vi "Enter_temp_sub_panel.vi"() -> ()   [LabVIEW 2011]
panel:
  in  "Stop":bool
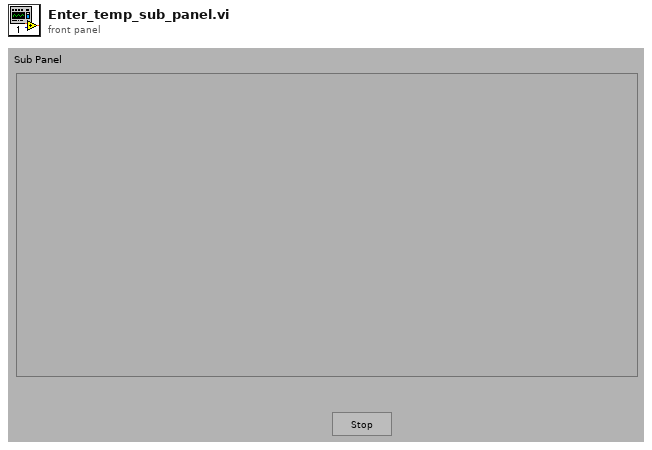
[diagram p1: front panel]
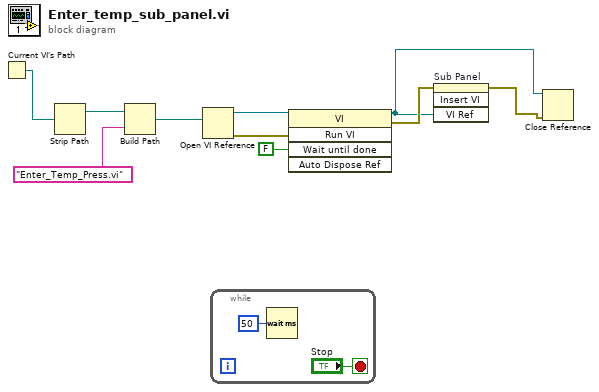
[diagram p0: block diagram]
diagram:
  n1 = Current VI's Path() -> (path=w10:path)
  n2 = Strip Path(path=w10) -> (stripped path=w9:path)  [unwired: 1 out]
  n3 = Build Path(base path=w9, name or relative path="Enter_Temp_Press.vi") -> (appended path=w7:path)
  n4 = Open VI Reference(vi path=w7) -> (vi reference=w5:refnum<vi>, error out=w4:errorcluster)  [unwired: 1 in, 4 out]
  n5 = while {
    stop <- "Stop" stop-if-true
    n6 = Wait (ms)(milliseconds to wait=u32 50) -> ()  [unwired: 1 out]
  }
  n7 = invoke class="VI" method="Run VI"(reference=w5, error in=w4, "Wait until done"=FALSE) -> (reference out=w1:refnum<vi>, error out=w3:errorcluster)  [unwired: 2 in, 3 out]
  n8 = invoke on="Sub Panel" class="SubPanel" method="Insert VI"(error in=w3, "VI Ref"=w1) -> (error out=w2:errorcluster)  [unwired: 2 in, 3 out]
  n9 = Close Reference(reference=w1, error in (no error)=w2) -> ()  [unwired: 1 out]
